vi "IMAQ FPGA FIFO to Pixel Bus HSL32x8.vi"(6 "Ready For Output":bool=TRUE, 10 "Image Size":T2, 11 "Source Image FIFO":refnum<k21>) -> (0 "Output Valid":bool, 2 "Source FIFO Status":T1, 3 "Pixel Bus Out":T3={"Pixel Data"={"A"=[0, 0, 0, 0, 0, 0, 0, 0], "R/H"=[0, 0, 0, 0, 0, 0, 0, 0], "G/S"=[0, 0, 0, 0, 0, 0, 0, 0], "B/L"=[0, 0, 0, 0, 0, 0, 0, 0]}, "DV"=[FALSE, FALSE, FALSE, FALSE, FALSE, FALSE, FALSE, FALSE], "EOL"=FALSE, "EOI"=FALSE, "Data Type"=enum."HSL32 x 8"})   [LabVIEW 2020, in "NI_VDM_FPGA_Basics.lvlib"]
doc: "Reads image pixels out of the specified FIFO and returns a Pixel Bus cluster of the requested type. The Pixel Bus contains the pixel data from the FIFO along with some additional flags that indicate when the pixel data is valid, an end of a line has been reached, or an end of the image has been reached. The Pixel Bus is used to pass image data to all of the other VIs in the NI Vision Development Module for FPGA library. Only one of the DV, EOL, and EOI flags in the Pixel Bus cluster will assert on a given clock cycle. When the last pixel of an image is reached, the Pixel Bus will contain the pixel data and the DV flag will be TRUE and the EOL and EOI flags will be FALSE. The next clock cycle, the EOL flag will be TRUE and the DV and EOI flags will be FALSE. The following clock cycle, the EOI flag will be TRUE and the DV and EOL flags will be FALSE."
uses:
  <vilib>/visionFPGA/NI_VDM_FPGA_Basics.lvlib
  <vilib>/rvi/DataTransferAndStorage/Container/XNode/niFpgaContainer.xnode
  <vilib>/visionFPGA/Controls/IMAQ FPGA Source FIFO Status.ctl
  <vilib>/visionFPGA/Controls/IMAQ FPGA Pixel Bus HSL32x8.ctl
  <vilib>/rvi/FIFO/Fifo_Resource/niFpgaFifoEmulationRefInMultiElement.vi
  <vilib>/visionFPGA/Controls/IMAQ FPGA Image Size.ctl
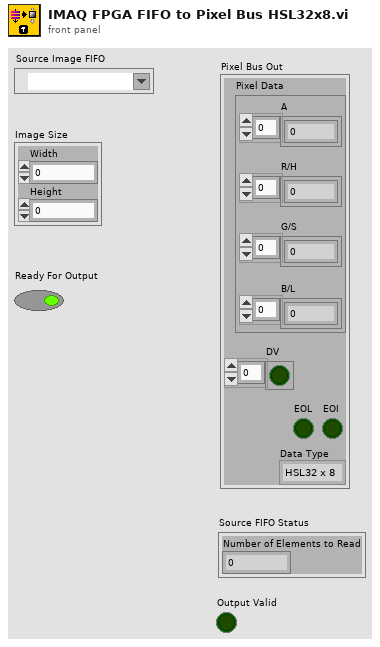
[diagram p1: front panel]
types:
  T1 = typedef "IMAQ FPGA Source FIFO Status.ctl" = cluster{"Number of Elements to Read":u32}
  T2 = typedef "IMAQ FPGA Image Size.ctl" = cluster{"Width":u32, "Height":u32}
  T3 = typedef "IMAQ FPGA Pixel Bus HSL32x8.ctl" = cluster{"Pixel Data":cluster{"A":u8[], "R/H":u8[], "G/S":u8[], "B/L":u8[]}, "DV":bool[], "EOL":bool, "EOI":bool, "Data Type":enum16{"HSL32 x 8"}}
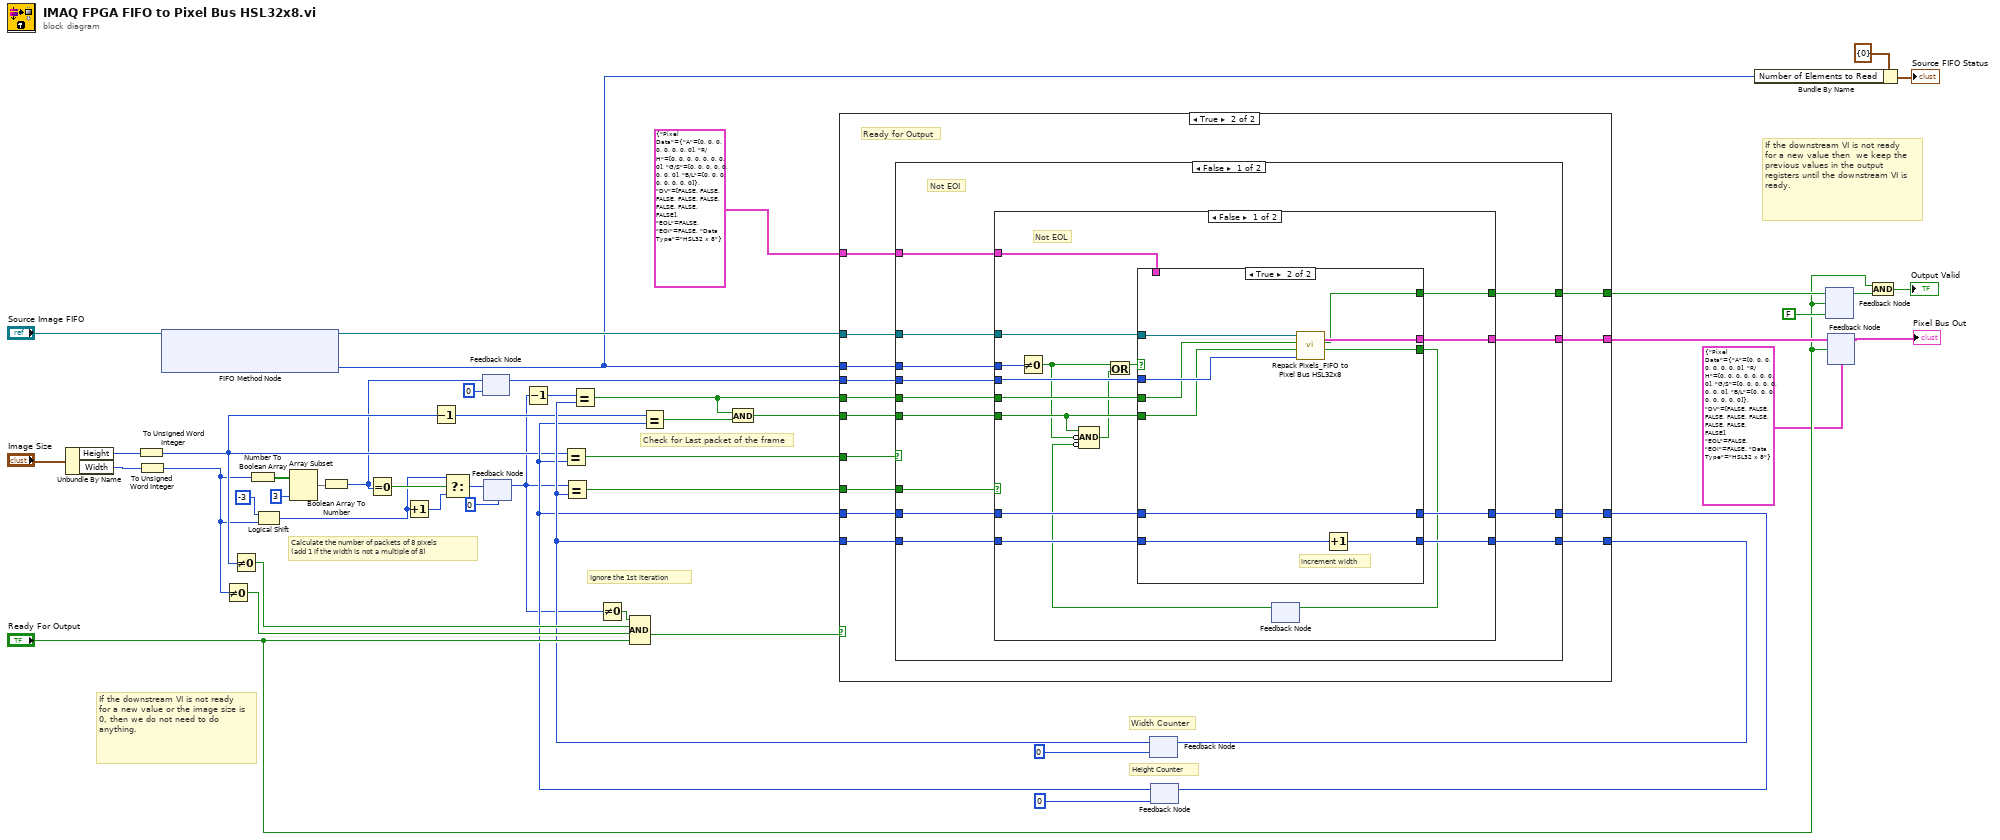
[diagram p0: block diagram]
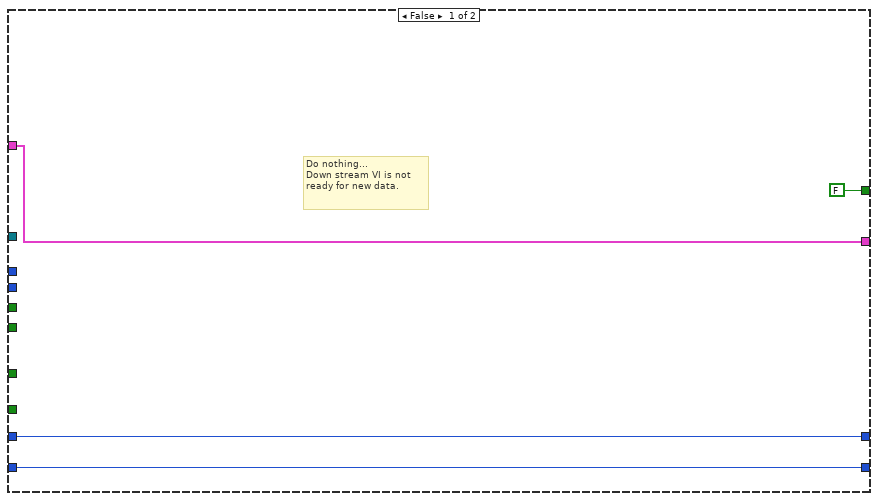
[diagram p2: hidden frame]
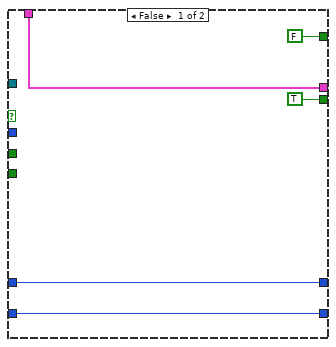
[diagram p3: hidden frame]
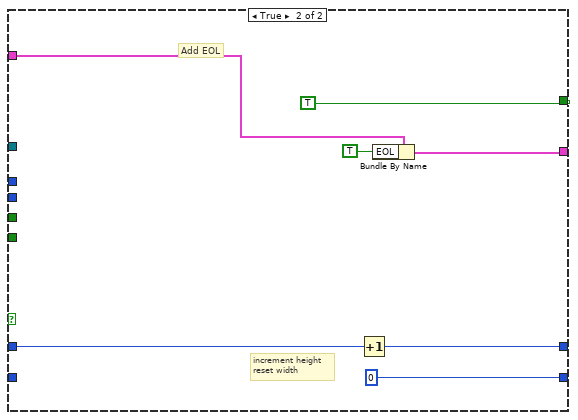
[diagram p4: hidden frame]
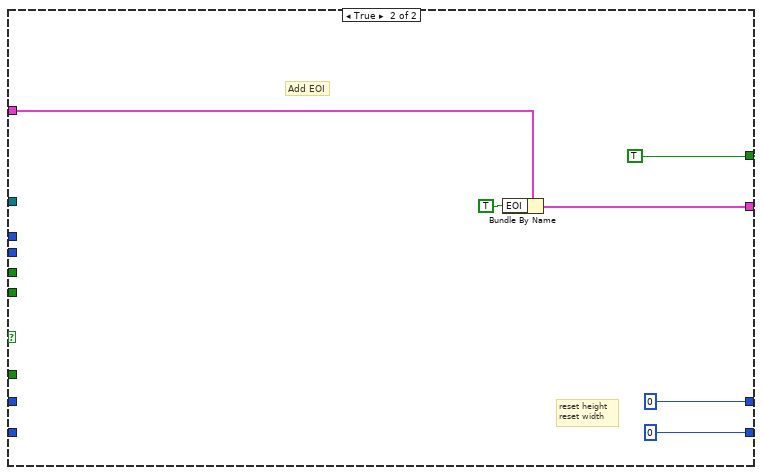
[diagram p5: hidden frame]
diagram:
  # "Ignore the 1st iteration"
  # "Calculate the number of packets of 8 pixels\n(add 1 if the width is not a multiple of 8)"
  # "Check for Last packet of the frame"
  # "If the downstream VI is not ready for a new value then  we keep the previous values in the output registers until the downstream VI is ready."
  # "If the downstream VI is not ready for a new value or the image size is 0, then we do not need to do anything."
  # "Height Counter"
  # "Width Counter"
  n1 = Unbundle By Name("Image Size") -> ("Height"=w20:u32, "Width"=w30:u32)
  n2 = To Unsigned Word Integer(number=w20) -> (unsigned 16bit integer=w15:u16)
  n3 = To Unsigned Word Integer(number=w30) -> (unsigned 16bit integer=w7:u16)
  n4 = xnode ("FIFO Method Node")("FIFO In"="Source Image FIFO") -> ("Number of Elements to Read"=w1:u32, "FIFO Out"=w2:refnum<k21>)
  n5 = Not Equal To 0?(x=w7) -> (x != 0?=w40:bool)
  n6 = Not Equal To 0?(x=w15) -> (x != 0?=w39:bool)
  n7 = Number To Boolean Array(number=w7) -> (Boolean array=w10:bool[])
  n8 = Logical Shift(y=i16 -3, x=w7) -> (x << y=w26:u16)
  n9 = Array Subset(array=w10, length=3) -> (w9:bool[])  [unwired: 1 in]
  n10 = Boolean Array To Number(Boolean array=w9) -> (number=w6:u8)
  n11 = Equal To 0?(x=w6) -> (x = 0?=w29:bool)
  n12 = Increment(x=w26) -> (x+1=w28:u16)
  n13 = Decrement(x=w15) -> (x-1=w21:u16)
  n14 = Select(t=w26, s=w29, f=w28) -> (s? t:f=w14:u16)
  n15 = feedback #1(u8 0) -> (w13:u8)
  n16 = feedback-in #1(w6) -> ()
  n17 = feedback #2(u16 0) -> (w4:u16)
  n18 = feedback-in #2(w14) -> ()
  n19 = Decrement(x=w4) -> (x-1=w24:u16)
  n20 = Not Equal To 0?(x=w4) -> (x != 0?=w5:bool)
  n21 = Compound Arithmetic op=AND(w5, w39, w40, "Ready For Output") -> (w41:bool)
  n22 = feedback #3(u16 0 ("Image Width")) -> (w25:u16)
  n23 = Equal?(x=w4, y=w25) -> (x = y?=w48:bool)
  n24 = Equal?(x=w24, y=w25) -> (x = y?=w17:bool)
  n25 = feedback #4(u16 0 ("Image Width")) -> (w19:u16)
  n26 = Equal?(x=w15, y=w19) -> (x = y?=w49:bool)
  n27 = Equal?(x=w21, y=w19) -> (x = y?=w18:bool)
  n28 = And(x=w17, y=w18) -> (x .and. y?=w16:bool)
  n29 = case shown="True" w41 {
    tunnel: w49 -> [_ w67]
    tunnel: T3 {"Pixel Data"={"A"=[0, 0, 0, 0, 0, 0, 0, 0], "R/H"=[0, 0, 0, 0, 0, 0, 0, 0], "G/S"=[0, 0, 0, 0, 0, 0, 0, 0], "B/L"=[0, 0, 0, 0, 0, 0, 0, 0]}, "DV"=[FALSE, FALSE, FALSE, FALSE, FALSE, FALSE, FALSE, FALSE], "EOL"=FALSE, "EOI"=FALSE, "Data Type"=enum."HSL32 x 8"} ("Pixel Bus Out 2") -> [w51 w66]
    tunnel: w48 -> [_ w65]
    tunnel: w1 -> [_ w64]
    tunnel: [FALSE ("EOI") w63] -> w47
    tunnel: [w52 w62] -> w45
    tunnel: w25 -> [w52 w61]
    tunnel: [w53 w60] -> w43
    tunnel: w19 -> [w53 w59]
    tunnel: [w51 w58] -> w42
    tunnel: w2 -> [_ w57]
    tunnel: w13 -> [_ w56]
    tunnel: w17 -> [_ w55]
    tunnel: w16 -> [_ w54]
    frame False {
      # "Do nothing...\nDown stream VI is not ready for new data."
    }
    frame True {
      # "Ready for Output"
      n30 = case shown="False" w67 {
        tunnel: w65 -> [w80 _]
        tunnel: [w79 TRUE ("EOI")] -> w63
        tunnel: [w78 w121] -> w58
        tunnel: w59 -> [w77 _]
        tunnel: w61 -> [w76 _]
        tunnel: [w75 u16 0 ("Height Counter")] -> w60
        tunnel: [w74 u16 0 ("Width Counter")] -> w62
        tunnel: w64 -> [w73 _]
        tunnel: w66 -> [w72 w120]
        tunnel: w57 -> [w71 _]
        tunnel: w56 -> [w70 _]
        tunnel: w55 -> [w69 _]
        tunnel: w54 -> [w68 _]
        frame False {
          # "Not EOI"
          n31 = case shown="False" w80 {
            tunnel: [w92 w118] -> w78
            tunnel: [w90 TRUE ("EOI")] -> w79
            tunnel: w77 -> [w87 w116]
            tunnel: w76 -> [w96 _]
            tunnel: [w88 w114] -> w75
            tunnel: [w95 u16 0 ("Width Counter")] -> w74
            tunnel: w73 -> [w97 _]
            tunnel: w72 -> [w89 w113]
            tunnel: w71 -> [w94 _]
            tunnel: w70 -> [w93 _]
            tunnel: w69 -> [w91 _]
            tunnel: w68 -> [w85 _]
            frame False {
              # "Not EOL"
              n32 = Not Equal To 0?(x=w97) -> (x != 0?=w84:bool)
              n33 = feedback #5() -> (w82:bool)  [unwired: 1 in]
              n34 = Compound Arithmetic op=AND(w85, invert w84, invert w82) -> (w81:bool)
              n35 = Or(x=w84, y=w81) -> (x .or. y?=w86:bool)
              n36 = case shown="True" w86 {
                tunnel: w96 -> [w100 w112]
                tunnel: [w100 w111] -> w95
                tunnel: w94 -> [_ w110]
                tunnel: w93 -> [_ w109]
                tunnel: [w101 w108] -> w92
                tunnel: w91 -> [_ w107]
                tunnel: [FALSE ("DV Out") w106] -> w90
                tunnel: w85 -> [_ w105]
                tunnel: w89 -> [w101 _]
                tunnel: [w99 w104] -> w88
                tunnel: w87 -> [w99 w104]
                tunnel: [TRUE ("Read/No Read") w103] -> w83
                frame False {
                }
                frame True {
                  # "increment width"
                  n37 = call <vilib>:"Repack Pixels_FIFO to Pixel Bus HSL32x8.vi"("Last \npacket length"=w109, "Last valid \npacket - Image"=w105, "Last valid \npacket - Row"=w107, "Source Image FIFO"=w110) -> ("Read/No Read"=w103:bool, "DV Out"=w106:bool, "Pixel Bus Out"=w108:T3)  [unwired: 5 in]
                  n38 = Increment(x=w112) -> (x+1=w111:u16)
                }
              }
              n39 = feedback-in #5(w83) -> ()
            }
            frame True {
              # "increment height\nreset width"
              # "Add EOL"
              n40 = Increment(x=w116) -> (x+1=w114:u16)
              n41 = Bundle By Name(cluster=w113, "EOL"=TRUE) -> (w118:T3)
            }
          }
        }
        frame True {
          # "reset height\nreset width"
          # "Add EOI"
          n42 = Bundle By Name(cluster=w120, "EOI"=TRUE) -> (w121:T3)
        }
      }
    }
  }
  n43 = feedback-in #3(w45) -> ()
  n44 = feedback-in #4(w43) -> ()
  n45 = Bundle By Name(cluster=T1 {"Number of Elements to Read"=0} ("FIFO Status"), "Number of Elements to Read"=w1) -> (→"Source FIFO Status":T1)
  n46 = feedback-in #6(w47, "Ready For Output") -> ()
  n47 = feedback #6(FALSE ("EOI")) -> (w37:bool)
  n48 = feedback-in #7(w42, "Ready For Output") -> ()
  n49 = feedback #7(T3 {"Pixel Data"={"A"=[0, 0, 0, 0, 0, 0, 0, 0], "R/H"=[0, 0, 0, 0, 0, 0, 0, 0], "G/S"=[0, 0, 0, 0, 0, 0, 0, 0], "B/L"=[0, 0, 0, 0, 0, 0, 0, 0]}, "DV"=[FALSE, FALSE, FALSE, FALSE, FALSE, FALSE, FALSE, FALSE], "EOL"=FALSE, "EOI"=FALSE, "Data Type"=enum."HSL32 x 8"} ("Pixel Bus Out 2")) -> (→"Pixel Bus Out":T3)
  n50 = And(x="Ready For Output", y=w37) -> (x .and. y?=→"Output Valid":bool)
